vi "Test View Broadcast When View is Shown.vi"(8 "error in (no error)":errorcluster, 11 "UI View Test In":refnum<class "View Test.lvclass">) -> (0 "error out":errorcluster, 3 "UI View Test Out":refnum<class "View Test.lvclass">)   [LabVIEW 2020, in "View Test.lvclass"]
uses:
  View Test.lvclass
  C:/Program Files (x86)/National Instruments/LabVIEW 2020/vi.lib/Asteme/LUnit/Test Case.lvclass
  Framework/Process/Process.lvclass/Process.ctl
  Framework/View/View.lvclass/View.ctl
  <vilib>/Asteme/LUnit/Test Case.lvclass/Test Case.ctl
  <vilib>/Asteme/LUnit/LUnit Assertion Result.lvclass/LUnit Assertion Result.ctl
  Support/Execution timer.vi
  Framework/Process/Protected/Messaging/Enqueue Message.vi
  Framework/View/Public/Get View VI Reference.vi
  Framework/Process/Public/Lifecycle/Get Lifecycle State.vi
  Framework/Process/Private/SubVIs/Wait for finish.vi
  Framework/Process/Private/SubVIs/Set Lifecycle State.vi
  <vilib>/Asteme/LUnit/Palette/Pass.vi
  <vilib>/Asteme/LUnit/Palette/Fail.vi
  <vilib>/Asteme/LUnit/Variant to string.vi
  <vilib>/Asteme/LUnit/Set Assertion Type.vi
  Framework/Process/Protected/Messaging/Request Message.vi
  <vilib>/Utility/error.llb/Clear Errors.vi
  <vilib>/Asteme/LUnit/Add test result.vi
  <vilib>/Asteme/LUnit/LUnit Write Passed.vi
  <vilib>/Asteme/LUnit/LUnit Get Test Case.vi
  <vilib>/Asteme/LUnit/Assertion Result/LUnit Get Test Name.vi
  <vilib>/Asteme/LUnit/LUnit Write Message.vi
  <vilib>/Asteme/LUnit/LUnit Write Description.vi
  <vilib>/Asteme/LUnit/LUnit Write Assertion Type.vi
  Framework/Process/Private/SubVIs/Enqueue Request Message.vi
  <vilib>/Asteme/LUnit/Read Test Case Name.vi
  Framework/View/View.lvclass
  C:/Users/anton/Documents/GitHub/Triarc-Framework/source/Framework/Process/Process.lvclass
  <vilib>/Utility/error.llb/Error Cluster From Error Code.vi
  Framework/Process/Private/SubVIs/Wait for Response Message.vi
  Support/Event Helpers/Dequeue Event Message.vi
  <vilib>/Utility/Data Type/Get Type Information.vi
  <vilib>/Utility/LVClass/Get LV Class Name.vi
  <vilib>/Asteme/LUnit/LUnit Assertion Result.lvclass
  Framework/Process/Process.lvclass
  Support/Event Helpers/Event Helpers.lvlib
  <vilib>/Asteme/LUnit/Test Case.lvclass
  C:/Users/anton/Documents/GitHub/Triarc-Framework/source/Framework/Base/Base.lvclass
  C:/Users/anton/Documents/GitHub/Triarc-Framework/source/Framework/Error Handler Interface/Error Handler Interface.lvclass
  C:/Users/anton/Documents/GitHub/Triarc-Framework/source/Framework/Logging/Logging.lvclass
  C:/Users/anton/Documents/GitHub/Triarc-Framework/source/Framework/View/View.lvclass
  C:/Users/anton/Documents/GitHub/Triarc-Framework/source/Framework Test/Process Test/Process Test.lvclass
  C:/Users/anton/Documents/GitHub/Triarc-Framework/source/Framework Test/Base Class Test/Base Test.lvclass
  C:/Users/anton/Documents/GitHub/Triarc-Framework/source/Framework Test/View Test/View Test.lvclass
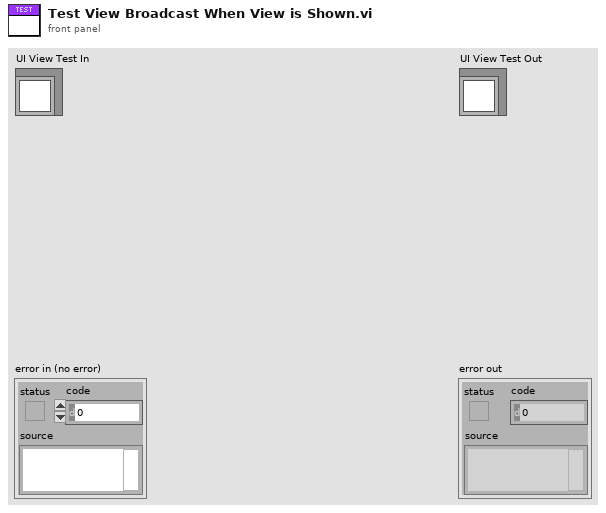
[diagram p1: front panel]
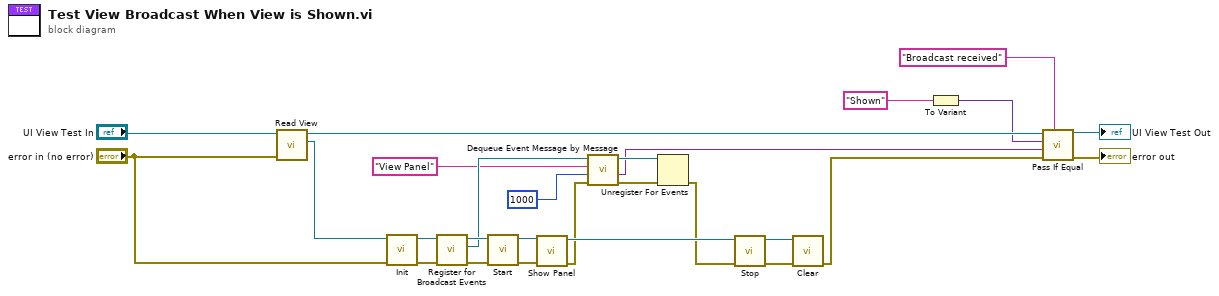
[diagram p0: block diagram]
diagram:
  n1 = call "Read View.vi"("error in (no error)"="error in (no error)", "View Test In"="UI View Test In") -> ("View"=w22:refnum<class "View.lvclass">, "View Test Out"=w25:refnum<class "View Test.lvclass">)  [unwired: 7 in, 1 out]
  n2 = call-dynamic "Init.vi"("error in (no error)"="error in (no error)", "View In"=w22) -> ("error out"=w17:errorcluster, "View Out"=w13:refnum<class "View.lvclass">)  [unwired: 8 in]
  n3 = call "Register for Broadcast Events.vi"("error in (no error)"=w17, "Process In"=w13) -> ("error out"=w14:errorcluster, "Event Registration Refnum Out"=w11:refnum<event-registration>, "Process Out"=w12:refnum<class "View.lvclass">)  [unwired: 7 in]
  n4 = call "Start.vi"("error in (no error)"=w14, "Process In"=w12) -> ("error out"=w20:errorcluster, "Process Out"=w21:refnum<class "View.lvclass">)  [unwired: 8 in]
  n5 = call "Show Panel.vi"("error in (no error)"=w20, "View In"=w21) -> ("error out"=w2:errorcluster, "View Out"=w15:refnum<class "View.lvclass">)  [unwired: 8 in]
  n6 = call "Dequeue Event Message by Message.vi"("error in (no error)"=w2, "Timeout (-1)"=1000, "Message"="View Panel", "Event Registration Refnum"=w11) -> ("error out"=w3:errorcluster, "Message Data"=w6:variant, "Event Registration Refnum Out"=w8:refnum<event-registration>)  [unwired: 3 in, 2 out]
  n7 = Unregister For Events(event registration refnum=w8, error in=w3) -> (error out=w1:errorcluster)
  n8 = call "Stop.vi"("error in (no error)"=w1, "Process In"=w15) -> ("error out"=w18:errorcluster, "Process Out"=w19:refnum<class "View.lvclass">)  [unwired: 7 in, 1 out]
  n9 = call-dynamic "Clear.vi"("error in (no error)"=w18, "View In"=w19) -> ("error out"=w7:errorcluster)  [unwired: 9 in]
  n10 = To Variant(anything="Shown") -> (Variant=w4:variant)
  n11 = call <vilib>:"Pass If Equal.vi"("Description"="Broadcast received", "error in (no error)"=w7, "Actual"=w6, "Expected"=w4, "Test Case In"=w25) -> ("error out"=→"error out":errorcluster, "Test Case Out"=→"UI View Test Out":refnum<class "View Test.lvclass">)  [unwired: 5 in]
